vi "OLD_Dashboard Main_Fixed_1280x768.vi"() -> ()   [LabVIEW 2023]
uses:
  <vilib>/Rock Robotics/WPI/ThirdParty/JAS_Junk/TrajLib/TypeDef/FieldDisp_ElementPicture.ctl
  <vilib>/event_ctls.llb/eventvkey.ctl
  <vilib>/Rock Robotics/WPI/ThirdParty/JAS_Junk/TrajLib/Rotation2d_CreateAngle.vi
  <vilib>/Rock Robotics/WPI/ThirdParty/JAS_Junk/TrajLib/Translation2d_Create.vi
  <vilib>/Rock Robotics/WPI/ThirdParty/JAS_Junk/TrajLib/VI/FieldDisp_Element_Rotate.vi
  <vilib>/Rock Robotics/WPI/ThirdParty/JAS_Junk/TrajLib/Conv_Meters_Inches.vi
  <vilib>/Rock Robotics/WPI/ThirdParty/JAS_Junk/TrajLib/Conv_Radians_Deg.vi
  <vilib>/Rock Robotics/WPI/Dashboard/WPI_DashboardLogging Global.vi
  <vilib>/Rock Robotics/Network Tables/NT Read Boolean.vi
  <vilib>/Rock Robotics/Network Tables/NT Write Boolean.vi
  <vilib>/picture/pixmap.llb/Flatten Pixmap.vi
  <vilib>/picture/pictutil.llb/Create Mask.vi
  <vilib>/picture/picture.llb/Draw Flattened Pixmap.vi
  <vilib>/Rock Robotics/WPI/ThirdParty/JAS_Junk/TrajLib/Trajectory_Library.lvlib
panel:
  out "ROBOT":T1
  in  "Camera Settings Right":T2={"Frame Rate"=30, "Compression"=30, "Size"=1, "DB Camera Config"=FALSE} {"Frame Rate" scale=1.0..30.0; "Compression" scale=100.0..-1.0; "Size" items=["640x480", "320x240", "160x120"]}
  in  "Camera Name Right":string(combo)="No Camera Selection"
  out "Camera Perf":string
  in  "Camera Settings":T2={"Frame Rate"=30, "Compression"=30, "Size"=1, "DB Camera Config"=FALSE} {"Frame Rate" scale=1.0..30.0; "Compression" scale=100.0..-1.0; "Size" items=["640x480", "320x240", "160x120"]}
  in  "TCP":refnum<k5>
  in  "Rec Mode":enum32{"Stop", "Record", "Playback"}(radio)
  out "Robot IP":string
  out "Image Message":string="Timeout in Camera Communications"
  in  "Dashboard Tab":T3(tab)
  out "Auto Arm":bool
  out "Lower Limit Switch":bool
  out "Right Limit":bool
  out "Left Limit":bool
  out "Position":dbl
  out "Demand":dbl
  out "On Target":bool
  in  "Intake Update":bool
  in  "Shoot Update":bool
  in  "Intake":dbl
  in  "Shoot Speed":dbl
  out "State":string
  out "Misaligned":bool
  out "Have Note":bool
  out "Box Ready":bool
  out "Selected Auto":string
  out "Int Gyro Feedback":dbl
  out "Int Gyro":dbl
  in  "Update":bool
  in  "Rotation":dbl
  out "Calibrated":bool
  in  "Calibrate":bool
  in  "Select Auto":string(combo)="Select Autonomous ..."
  out "NT Connection":bool
  out "JS1 Z":dbl(slide) scale=-1.0..1.0 scale format="%#_2e"
  out "JS1 Graph":cluster{"X":dbl, "Y":dbl}[](graph)
  out "JS1 Buttons":T4
  out "JS2 Z":dbl(slide) scale=-1.0..1.0 scale format="%#_2e"
  out "JS2 Graph":cluster{"X":dbl, "Y":dbl}[](graph)
  out "JS2 Buttons":T4
  out "Mode":T5(ring)=enum."Auto Disabled"
  out "Right Camera Perf":cluster{"Bandwidth (Mbps)":dbl, "FPS":dbl}
  out "Camera Image Right":T6(plugin-control)
  out "Arm on Target":bool
  out "Velocity Deg/Sec":dbl format="%11.1f"
  out "CO":dbl format="%11.2f"
  out "PV Deg":dbl format="%11.1f"
  out "SP Deg":dbl format="%11.1f"
  out "Arm Chart":T7(graph)
  out "Right Vel":dbl format="%11.1f"
  out "Left Vel":dbl format="%11.1f"
  out "Right On Targ":bool
  out "Left On Targ":bool
  out "Right Upper (Virtual) Limit":bool
  out "Left Upper (Virtual) Limit":bool
  out "Right Low Limit":bool
  out "Right Co":dbl format="%11.2f"
  out "Right PV":dbl format="%11.1f"
  out "Left Co":dbl format="%11.2f"
  out "Left PV":dbl format="%11.1f"
  out "SP Inches":dbl format="%11.1f"
  out "Left Low Limit":bool
  out "Climb Chart":T8(graph)
  out "Left Pos":dbl
  out "Right Pos":dbl
  out "Dmd 2":dbl
  out "Right\nPosition":u8(slide) scale=0.0..14.0
  out "Left\nPosition":u8(slide) scale=0.0..14.0
  out "Dmd":u8(slide) scale=0.0..14.0
  out "Climb Blocked":bool
  out "L Mot":dbl format="%11.2f"
  out "L Speed":dbl format="%11.1f"
  out "R Mot":dbl format="%11.2f"
  out "R Speed":dbl format="%11.1f"
  out "Shoot SP\nRPM":dbl format="%11.1f"
  out "Shoot Chart":T8(graph)
  out "Robot Angle":dbl format="%11.1f"
  out "Robot Y":dbl format="%11.2f"
  out "Robot X":dbl format="%11.2f"
  out "Right April Tag Updated":bool
  out "Left April Tag Updated":bool
  out "Right Cam Connected":bool
  out "Left Cam Connected":bool
  out "Field Picture":picture
  in  "Test Slider":dbl(slide) scale=0.0..100.0 scale format="%#_3g"
  in  "On/Off":bool caption="Solenoid"
  in  "Test Name":u16(ring) items=["Select the test to run..."]
  in  "Test Tree":string(tree)
  in  "Motor":cluster{"Value":dbl, "Enable":bool} {"Value" scale=-1.0..1.0 scale format="%#_3g"}
  out "Progress":T9 {"Test Progress" scale=0.0..100.0}
  in  "Rev/Fwd":cluster{"Forward":bool, "Reverse":bool}
  in  "Test Ring":u16(ring) items=["Monochrome", "Color"]
  in  "CheckList":i32(listbox)
  out "Tree":string(tree)
  out "Camera Image":T6(plugin-control)
  in  "Camera Name":string(combo)="No Camera Selection"
  out "Background":bool
  # "HW"
  # "HW"
  # "Joysticks"
  # "Arm"
  # "Climb"
  # "Initial Rotation"
  # "Shooter & Intake"
  # "Box"
  # "Gyro"
  # "Auto"
  # "No Varible Written"
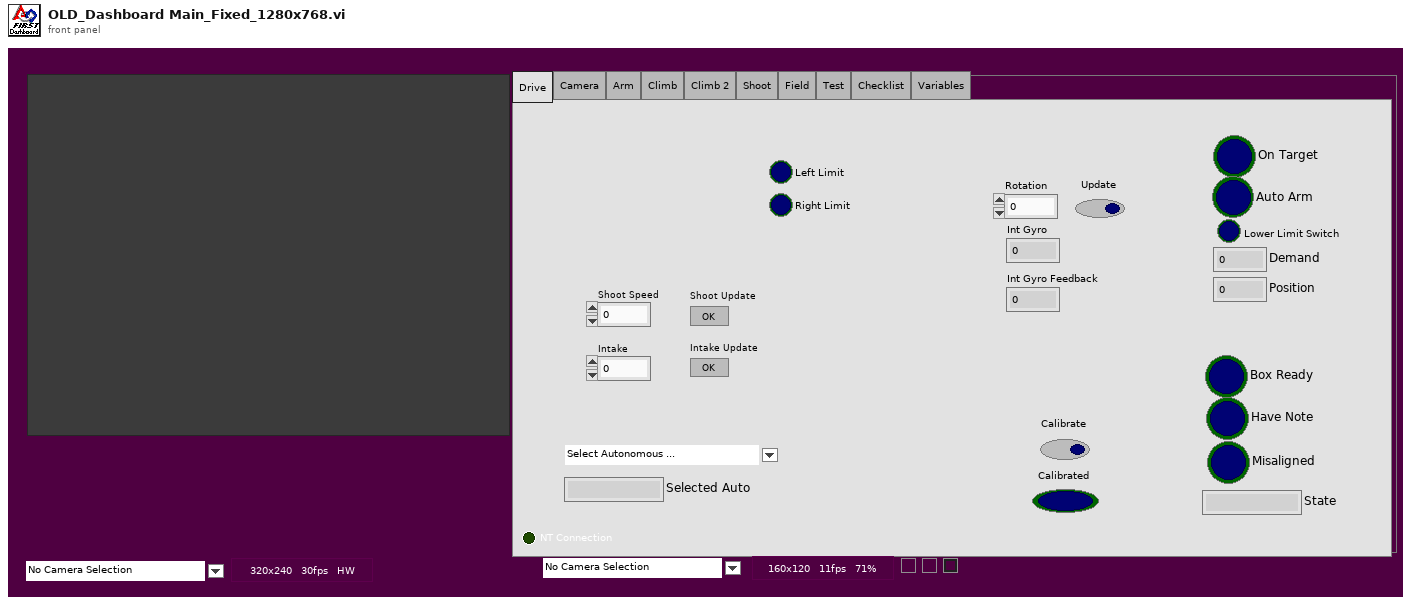
[diagram p1: front panel]
types:
  T1 = typedef "Trajectory_Library.lvlib/FieldDisp_ElementPicture.ctl" = picture
  T2 = cluster{"Frame Rate":i32, "Compression":i32, "Size":u16, "DB Camera Config":bool}
  T3 = enum32{"Drive", "Camera", "Arm", "Climb", "Climb 2", "Shoot", "Field", "Test", "Checklist", "Variables"}
  T4 = cluster{bool, bool, bool, bool, bool, bool, bool, bool, bool, bool, bool, bool}
  T5 = enum8{"Tele-Op Disabled", "Tele-Op Enabled", "Auto Disabled", "Auto Enabled", "Test Disabled", "Test Enabled", "Disconnected", "No Code", "E-Stop"}
  T6 = typedef "IMAQ Image.ctl" = refnum<image>
  T7 = cluster{"value":dbl, "value":dbl, "value":dbl, "value":dbl}
  T8 = cluster{"value":dbl, "value":dbl, "value":dbl, "value":dbl, "value":dbl}
  T9 = cluster{"Test Progress":u8, "Test Progress Text":string}
  T10 = cluster{"Save Path":path, "Interval (s)":dbl, "Keep":i32}
  T11 = enum32{"Drive", "Camera", "Basic", "Custom", "Test", "Commands", "Checklist", "Variables"}
  T12 = typedef "Image Type" = u32
  T13 = cluster{"Camera Image":refnum<vi>, "Dashboard Tab":refnum<vi>, "Background":refnum<vi>, "Rec Mode":refnum<vi>, "Test Slider":refnum<vi>, "On/Off ":refnum<vi>, "Test Ring":refnum<vi>, "Rev/Fwd":refnum<vi>, "Test Name":refnum<vi>, "Motor":refnum<vi>, "Progress":refnum<vi>, "CheckList":refnum<vi>, "Tree":refnum<vi>, "Test Tree":refnum<vi>, "Camera Settings":refnum<vi>, "Camera Name":refnum<vi>, "Camera Perf":refnum<vi>, "Camera Settings Right":refnum<vi>, "Camera Name Right":refnum<vi>, "Camera Image Right":refnum<vi>}
  T14 = cluster{"Global Rectangle":i32[], "Contours":cluster{"Contour Type":u32, "ROI Type":u32, "Points":i32[]}[]}
  T15 = cluster{"Camera Name":string, string, "Saved DB Images Info":cluster{"Save Path":path, "Interval (s)":dbl, "Keep":i32}}
  T16 = cluster{"Camera Name Right":string, string, "Saved DB Images Info":cluster{"Save Path":path, "Interval (s)":dbl, "Keep":i32}}
  T17 = cluster{"Operation":enum16{"Update", "Clear"}, "Color Box":u32}[]
  T18 = typedef "eventvkey.ctl" = enum16{"ASCII", "Enter", "Return", "Shift", "Ctrl", "Alt", "Cmd", "Opt", "Caps", "NumLock", "Clear", "Break", "Up", "Down", "Left", "Right", "Insert", "Delete", "Home", "End", "PageUp", "PageDown", "Escape", "Help", "Pause", "ScrollLock", "F1", "F2", "F3", "F4", "F5", "F6", "F7", "F8", "F9", "F10", "F11", "F12", "F13", "F14", "F15", "F16", "F17", "F18", "F19", "F20", "F21", "F22", "F23", "F24", "Play", "VolumeUp", "VolumeDown", "Mute", "Two Byte Char"}
  T19 = cluster{"Image Size":bool, "Image Type":bool, "Pixel Value":bool, "ROI Information":bool, "Zoom Factor":bool}
  T20 = cluster{"Operation":enum16{"Update", "Clear"}, "Color Box":u32}
  T21 = cluster{"Shift":bool, "Ctrl":bool, "Alt":bool, "Cmd":bool, "Opt":bool}
  T22 = typedef "Trajectory_Library.lvlib/FieldDisp_FieldElement.ctl" = cluster{"ONE-8-bit pixmap":u8[][], "Two-Array":cdb[][], "Three-Numeric":i32, "Four-Numeric":i32, "Five-Numeric":cdb, "Six-colors":u32[], "Seven-new element/subarray":u32, "Left Pixel":dbl, "Top Pixel":dbl, "Width Pix/Ft":dbl, "Height Pix/Ft":dbl, "Element Picture Ref":refnum<vi>}
  T23 = enum32{"Drive", "Camera", "Box", "Arm", "Arm 2", "Climb", "Climb 2", "Shoot", "Auto", "Field", "Vision", "Test", "Checklist", "Variables"}
  T24 = cluster{"Error Strings":string, "Disable Counts":cluster{u16, u16}, "Rail Faults":cluster{u16, u16, u16}, "Robot IP":string, "DB Mode":u8, "Event Info":cluster{"Name":string, "Type":u8, "Number":u16, "Replay":u8}}
  T25 = cluster{"Storage":cluster{"Disk Free":u64, "RAM Block":u32, "RAM free":u32}, "CPU Utilization":cluster{"CPU % ISR":sgl, "CPU % Time Crit":sgl, "CPU % Timed Str":sgl, "CPU % High":sgl, "CPU % Above":sgl, "CPU % Normal":sgl, "CPU % Low":sgl}, "CAN":cluster{"% Bus Utilization":sgl, "Bus Off Cnt":u32, "TX_FIFO Full Cnt":u32, "Receive Error Cnt":u8, "Transmit Error Cnt":u8}, "HID":cluster{"HID Outputs":u32, "Rumble Low":u16, "Rumble High":u16}[]}
  T26 = cluster{"Status bits":cluster{"Test Mode":bool, "Autonomous":bool, "Enabled":bool, "Code Start":bool, "Brownout":bool, "Reserved 2":bool, "Reserved 3":bool, "E-Stop":bool}, "Code Trace":cluster{"Disabled":bool, "TeleOp":bool, "Auto":bool, "Test":bool}, "Controller Type":enum16{"unknown", "cRIO", "roboRio"}, "Code?":enum16{"unknown", "noCode", "code"}, "Battery V":dbl}
  T27 = cluster{"Control Bits":cluster{"TestMode":bool, "Autonomous":bool, "Enabled":bool, "FMS Present":bool, bool, bool, bool, "E-Stop":bool}, "Team Station ":u8, "Countdown":sgl, "Joystick Values":cluster{"Axes":dbl[], "Buttons":bool[], "POVs":i16[]}[]}
  T28 = cluster{"Axes":dbl[], "Buttons":bool[], "POVs":i16[]}[]
  T29 = cluster{"Axes":dbl[], "Buttons":bool[], "POVs":i16[]}
  T30 = cluster{"Buttons[0]":bool, "Buttons[1]":bool, "Buttons[2]":bool, "Buttons[3]":bool, "Buttons[4]":bool, "Buttons[5]":bool, "Buttons[6]":bool, "Buttons[7]":bool, "Buttons[8]":bool, "Buttons[9]":bool, "Buttons[10]":bool, "Buttons[11]":bool}
  T31 = typedef "Trajectory_Library.lvlib/POSE2D.ctl" = cluster{"TRANSLATION":T32, "ROTATION":T33}
  T32 = typedef "Trajectory_Library.lvlib/TRANSLATION2D.ctl" = cluster{"X":dbl, "Y":dbl}
  T33 = typedef "Trajectory_Library.lvlib/ROTATION2D.ctl" = cluster{"VALUE":dbl, "COS":dbl, "SIN":dbl}
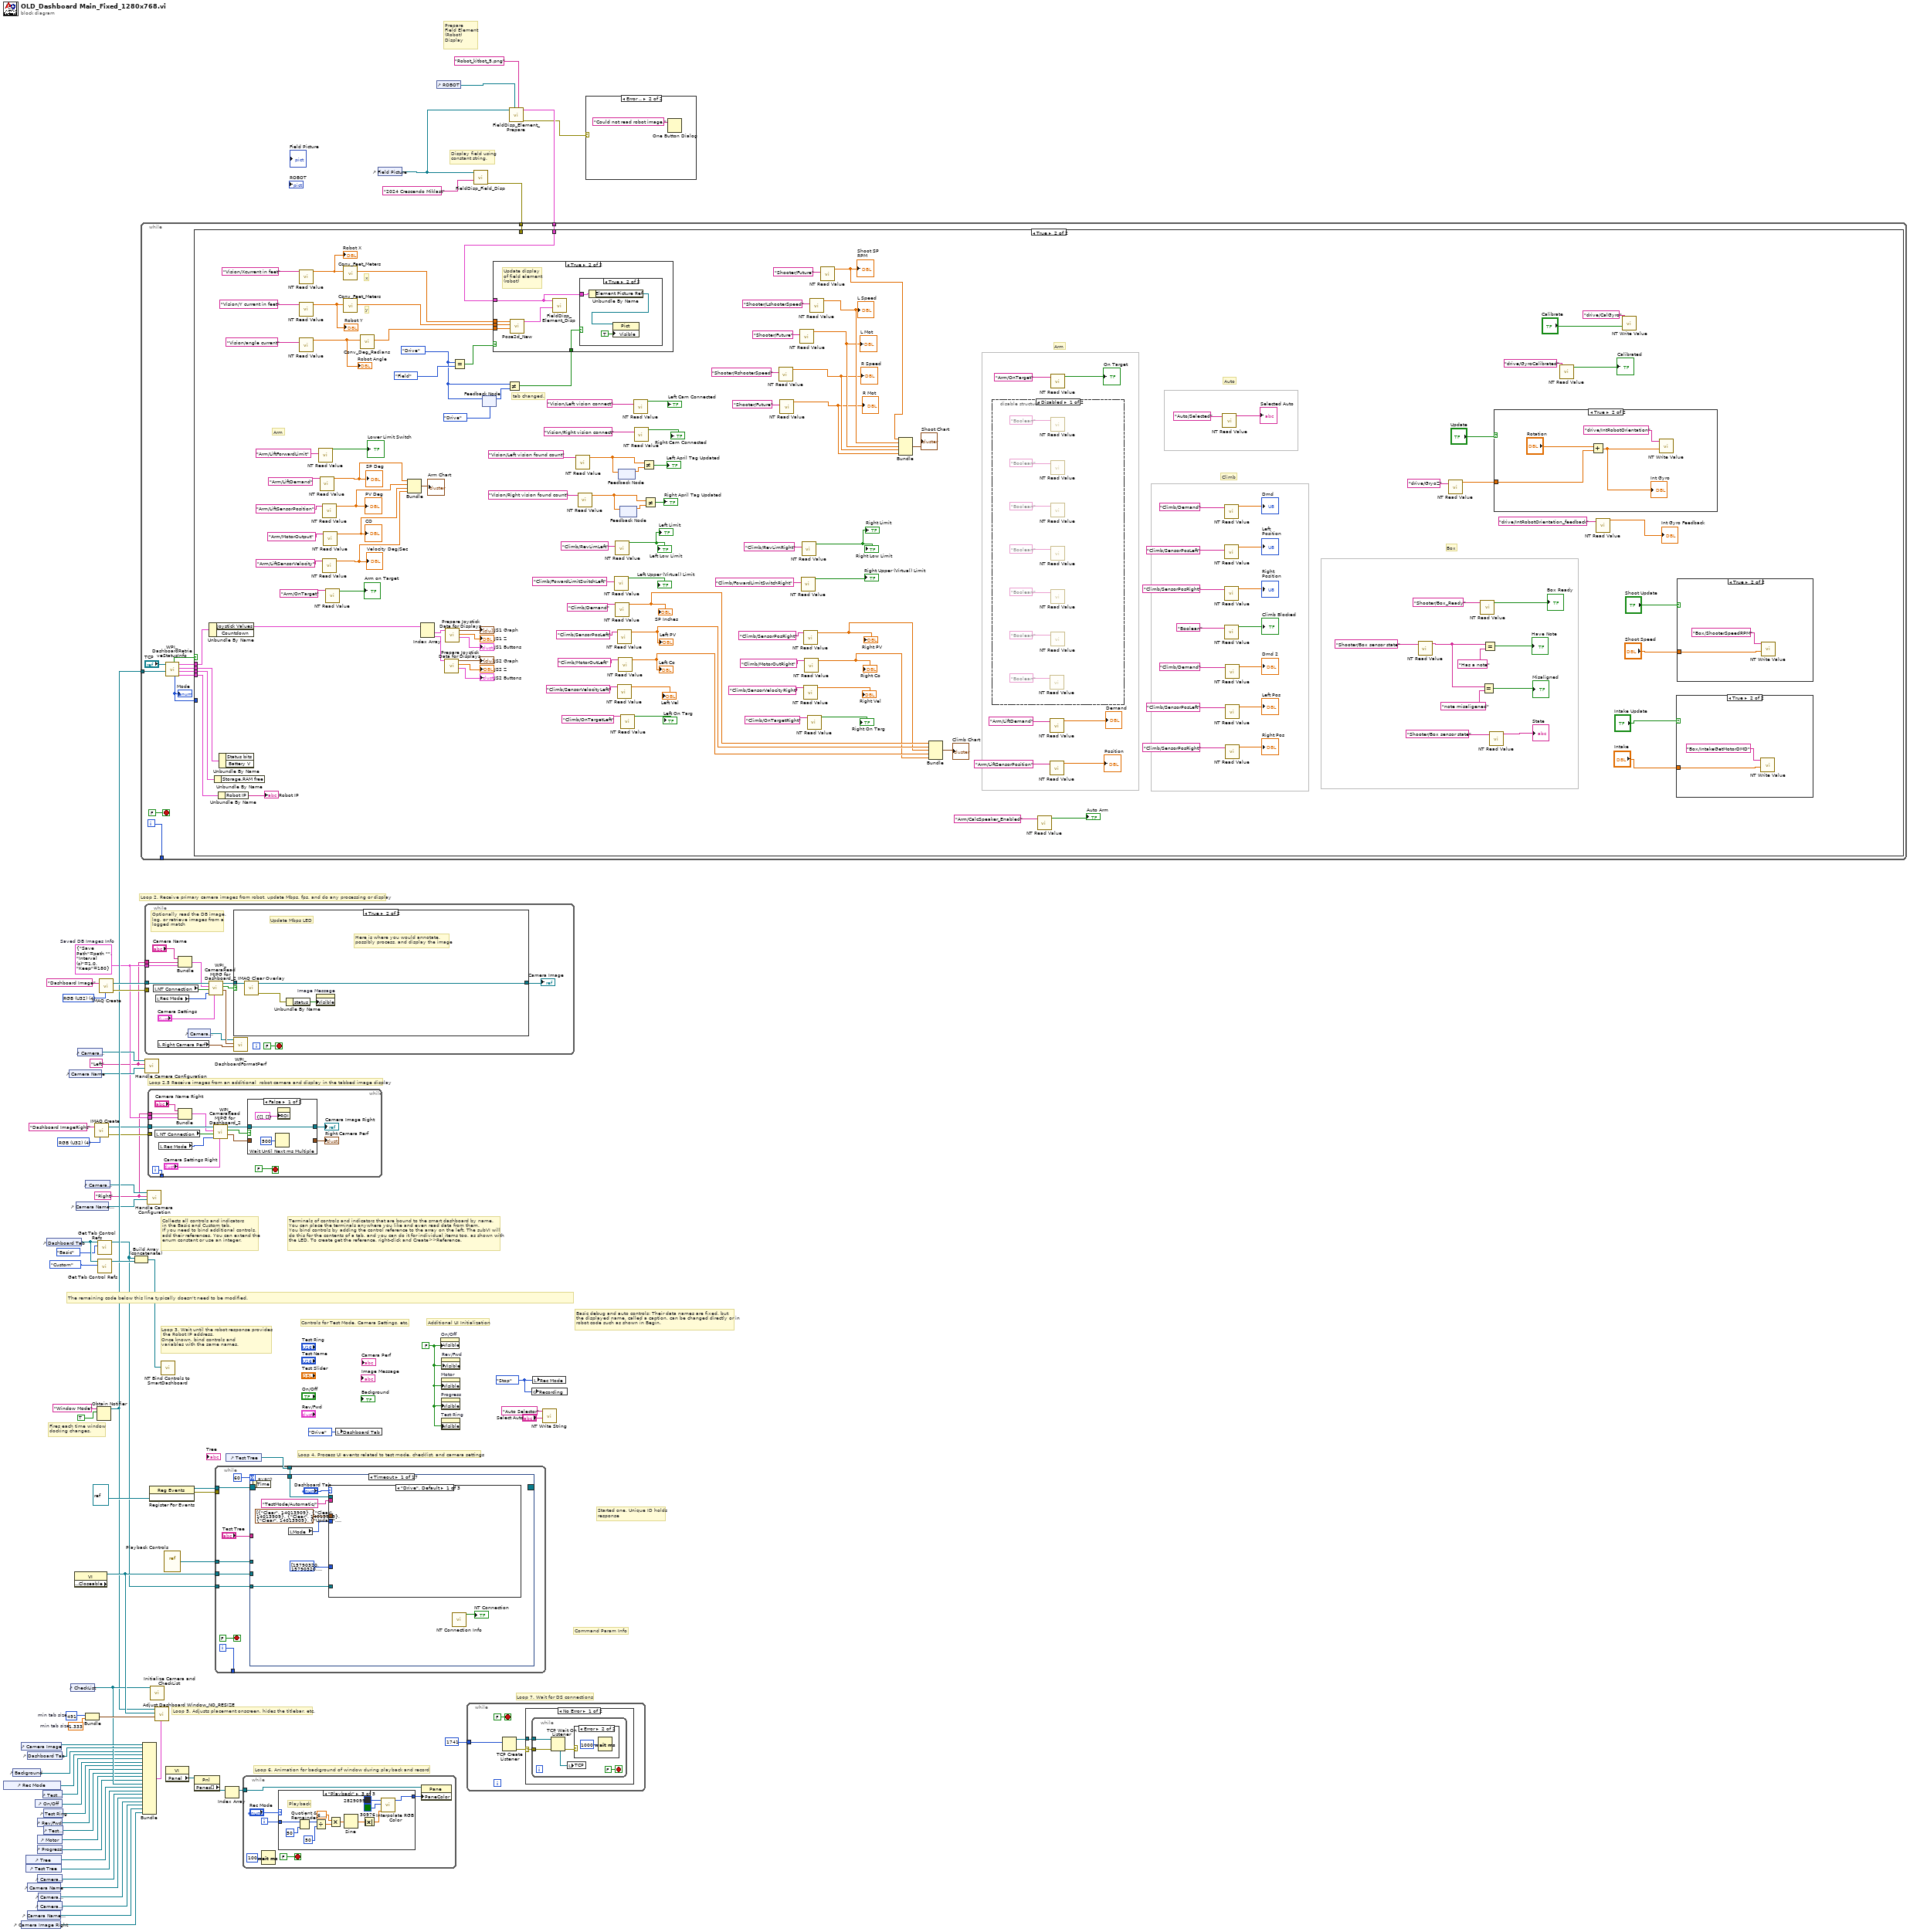
[diagram p0: block diagram]
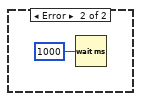
[diagram p5: hidden frame]
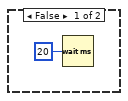
[diagram p6: hidden frame]
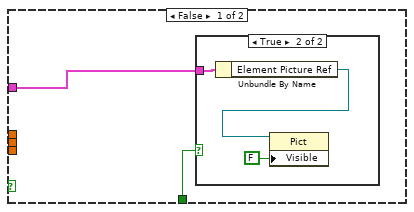
[diagram p11: hidden frame]
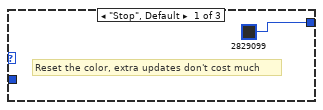
[diagram p14: hidden frame]
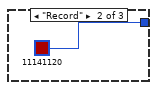
[diagram p15: hidden frame]
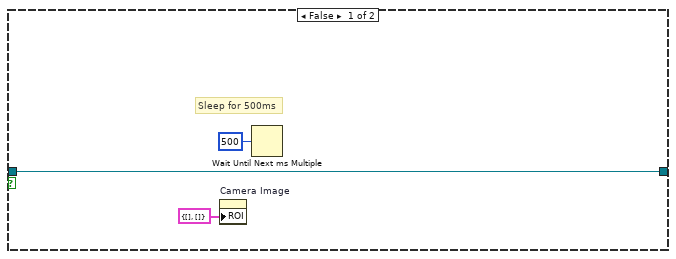
[diagram p16: hidden frame]
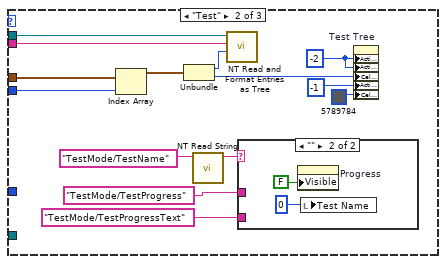
[diagram p17: hidden frame]
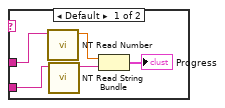
[diagram p18: hidden frame]
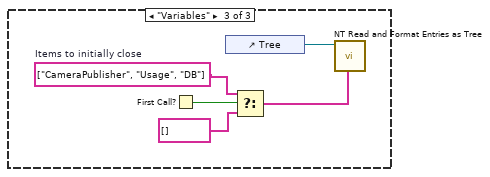
[diagram p19: hidden frame]
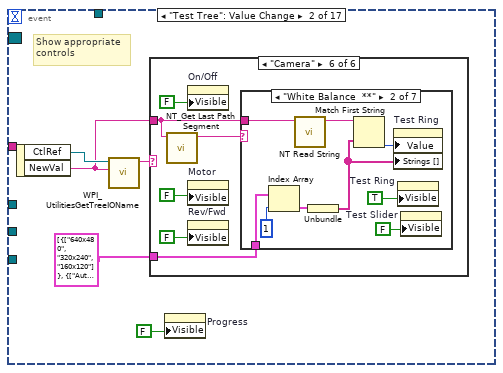
[diagram p20: hidden frame]
diagram:
  w12 = T10 {"Save Path"=path "", "Interval (s)"=1.0, "Keep"=180}  # Saved DB Images Info
  w11 = "Right"
  w10 = "Left"
  w22 = T12 4 items=["Grayscale (U8)", "Grayscale (I16)", "Grayscale (SGL)", "Complex (CSG)", "RGB (U32)", "HSL (U32)", "RGB (U64)"] ("Image Type")
  w49 = 491  # min tab size
  w48 = 1.333  # min tab size
  w56 = enum32{"Stop", "Record", "Playback"}."Stop" ("Rec Mode")
  w34 = FALSE ("Visible")
  w70 = T12 4 items=["Grayscale (U8)", "Grayscale (I16)", "Grayscale (SGL)", "Complex (CSG)", "RGB (U32)", "HSL (U32)", "RGB (U64)"] ("Image Type")
  # "Prepare\nField Element\n(Robot)\nDisplay"
  # "Display field using\nconstant string."
  # "Loop 2.5 Receive images from an additional  robot camera and display in the tabbed image display"
  # "Command Param Info"
  # "Started one, Unique ID holds\nresponse"
  # "Loop 7. Wait for DS connections"
  # "Basic debug and auto controls: Their data names are fixed, but\nthe displayed name, called a caption, can be changed directly or in\nrobot code such as shown in Begin."
  # "Controls for Test Mode, Camera Settings, etc."
  # "Additional UI Initialization"
  # "Loop 6. Animation for background of window during playback and record"
  # "Fires each time window\ndocking changes."
  # "Collects all controls and indicators\nin the Basic and Custom tab.\nIf you need to bind additional controls,\nadd their references. You can extend the\nenum constant or use an integer."
  # "The remaining code below this line typically doesn't need to be modified."
  # "Loop 4. Process UI events related to test mode, checklist, and camera settings"
  # "Terminals of controls and indicators that are bound to the smart dashboard by name.\nYou can place the terminals anywhere you like and even read data from them.\nYou bind controls by adding the control reference to the array on the left. The subVI will\ndo this for the contents of a tab, and you can do it for individual items too, as shown with\nthe LED. To create get the reference, right-click and Create>>Reference."
  # "Loop 3. Wait until the robot response provides\n the Robot IP address.\nOnce known, bind controls and\nvariables with the same names."
  # "Loop 5. Adjusts placement onscreen, hides the titlebar, etc."
  # "Loop 2. Receive primary camera images from robot, update Mbps, fps, and do any processing or display"
  n1 = control-ref of="Rec Mode"() -> (w40:refnum<vi>)
  n2 = control-ref of="Background"() -> (w9:refnum<vi>)
  n3 = control-ref of="Camera Image Right"() -> (w15:refnum<vi>)
  n4 = control-ref of="Camera Image"() -> (w51:refnum<vi>)
  n5 = control-ref of="Tree"() -> (w44:refnum<vi>)
  n6 = control-ref of="Test Tree"() -> (w43:refnum<vi>)
  n7 = control-ref of="Dashboard Tab"() -> (w50:refnum<vi>)
  n8 = control-ref of="Camera Name"() -> (w28:refnum<vi>)
  n9 = control-ref of="Camera Name Right"() -> (w16:refnum<vi>)
  n10 = control-ref of="On/Off"() -> (w38:refnum<vi>)
  n11 = control-ref of="Progress"() -> (w35:refnum<vi>)
  n12 = control-ref of="Camera Settings"() -> (w29:refnum<vi>)
  n13 = control-ref of="Camera Settings Right"() -> (w17:refnum<vi>)
  n14 = control-ref of="Rev/Fwd"() -> (w36:refnum<vi>)
  n15 = control-ref of="Motor"() -> (w41:refnum<vi>)
  n16 = control-ref of="Camera Perf"() -> (w27:refnum<vi>)
  n17 = control-ref of="Test Slider"() -> (w39:refnum<vi>)
  n18 = control-ref of="Test Ring"() -> (w37:refnum<vi>)
  n19 = control-ref of="Test Name"() -> (w42:refnum<vi>)
  n20 = control-ref of="Dashboard Tab"() -> (w54:refnum<vi>)
  n21 = control-ref of="Camera Name"() -> (w30:refnum<vi>)
  n22 = control-ref of="CheckList"() -> (w45:refnum<vi>)
  n23 = property class="VI" props=["Front Panel.Closeable"]() -> (reference out=w55:refnum<vi>)  [unwired: 2 in, 2 out]
  n24 = control-ref of="Camera Name Right"() -> (w18:refnum<vi>)
  n25 = control-ref of="Camera Settings"() -> (w31:refnum<vi>)
  n26 = control-ref of="Camera Settings Right"() -> (w19:refnum<vi>)
  n27 = Bundle("min tab size"=w49, "min tab size"=w48) -> (w47:cluster{"min tab size":i32, "min tab size":dbl})  [unwired: 1 in]
  n28 = call "IMAQ Create"("Image Name"="Dashboard ImageRight", "Image Type"=w22) -> ("New Image"=w21:T6, "error out"=w20:errorcluster)  [unwired: 2 in, 1 out]
  n29 = Obtain Notifier(name (unnamed)="Window Mode", notification data type=TRUE) -> (notifier out=w33:refnum<notifier>)  [unwired: 2 in, 2 out]
  n30 = call <vilib>:"Get Tab Control Refs.vi"("Page Index"=T11."Basic" ("Dashboard Tab"), "TabControl in"=w54) -> ("ControlsOnPage"=w26:refnum<vi>[])  [unwired: 9 in]
  n31 = call <vilib>:"Get Tab Control Refs.vi"("Page Index"=T11."Custom" ("Dashboard Tab"), "TabControl in"=w54) -> ("ControlsOnPage"=w53:refnum<vi>[])  [unwired: 9 in]
  n32 = call "IMAQ Create"("Image Name"="Dashboard Image", "Image Type"=w70) -> ("New Image"=w68:T6, "error out"=w67:errorcluster)  [unwired: 2 in, 1 out]
  n33 = Build Array (concatenate)(w26, w53) -> (w52:refnum<vi>[])
  n34 = Bundle("Camera Image"=w51, "Dashboard Tab"=w50, "Background"=w9, "Rec Mode"=w40, "Test Slider"=w39, "On/Off"=w38, "Test Ring"=w37, "Rev/Fwd"=w36, "Test Name"=w42, "Motor"=w41, "Progress"=w35, "CheckList"=w45, "Tree"=w44, "Test Tree"=w43, "Camera Settings"=w29, "Camera Name"=w28, "Camera Perf"=w27, "Camera Settings Right"=w17, "Camera Name Right"=w16, "Camera Image Right"=w15) -> (w46:T13)  [unwired: 1 in]
  n35 = call "Handle Camera Configuration.vi"("CameraNameRef"=w30, "Display Name"=w10, "ClusterRef"=w31) -> ()  [unwired: 9 in]
  n36 = while {
    tunnel: w68 -> [w84]
    tunnel: w67 -> [_]
    tunnel: w12 -> [w77]
    tunnel: w10 -> [w74]
    stop <- FALSE stop-if-true
    # "Optionally read the DB image,\nlog, or retrieve images from a\nlogged match"
    n37 = local read "NT Connection"() -> (w78:bool)
    n38 = local read "Rec Mode"() -> (w81:enum32{"Stop", "Record", "Playback"})
    n39 = local read "Right Camera Perf"() -> (w72:cluster{"Bandwidth (Mbps)":dbl, "FPS":dbl})
    n40 = Bundle("Camera Name"="Camera Name", w74, "Saved DB Images Info"=w77) -> (w76:T15)  [unwired: 1 in]
    n41 = control-ref of="Camera Perf"() -> (w71:refnum<vi>)
    n42 = call <vilib>:"WPI_CameraRead MJPG for Dashboard_2.vi"("Camera Settings"="Camera Settings", "Rec Mode"=w81, "NT Connection"=w78, "Capture Info"=w76, "Image in"=w84) -> ("perf info"=w73:cluster{"Bandwidth (Mbps)":dbl, "fps":dbl}, "Active"=w82:bool, "Image\\ out"=w83:T6)  [unwired: 4 in]
    n43 = case shown="True" w82 {
      tunnel: w83 -> [w87 w90]
      tunnel: [w87 w89] -> w79
      frame False {
        # "Sleep for 500ms"
        n44 = property on="Camera Image" class="ImageControl"("ROI"=T14 {"Global Rectangle"=[], "Contours"=[]}) -> ()  [unwired: 2 in, 2 out]
        n45 = Wait Until Next ms Multiple(millisecond multiple=u32 500) -> ()  [unwired: 1 out]
      }
      frame True {
        # "Here is where you would annotate,\npossibly process, and display the image"
        # "Update Mbps LED"
        n46 = call "IMAQ Clear Overlay"("Image"=w90) -> ("error out"=w91:errorcluster, "Image Out"=w89:T6)  [unwired: 2 in, 7 out]
        n47 = Unbundle By Name(w91) -> ("status"=w92:bool)
        n48 = property on="Image Message" class="Str"("Visible"=w92) -> ()  [unwired: 2 in, 2 out]
      }
    }
    "Camera Image" <- w79
    n49 = call <vilib>:"WPI_DashboardFormatPerf.vi"("Right Camera Perf"=w72, "Performance"=w73, "String in"=w71) -> ()  [unwired: 9 in]
  }
  n50 = call "Handle Camera Configuration.vi"("CameraNameRef"=w18, "Display Name"=w11, "ClusterRef"=w19) -> ()  [unwired: 9 in]
  n51 = while {
    tunnel: w21 -> [w107]
    tunnel: w20 -> [_]
    tunnel: [w102] -> _
    tunnel: w12 -> [w98]
    tunnel: w11 -> [w95]
    i -> [w102]
    stop <- FALSE stop-if-true
    n52 = local read "NT Connection"() -> (w99:bool)
    n53 = local read "Rec Mode"() -> (w106:enum32{"Stop", "Record", "Playback"})
    n54 = Bundle("Camera Name Right"="Camera Name Right", w95, "Saved DB Images Info"=w98) -> (w97:T16)  [unwired: 1 in]
    n55 = call <vilib>:"WPI_CameraRead MJPG for Dashboard_2.vi"("Camera Settings"="Camera Settings Right", "Rec Mode"=w106, "NT Connection"=w99, "Capture Info"=w97, "Image in"=w107) -> ("perf info"=w93:cluster{"Bandwidth (Mbps)":dbl, "fps":dbl}, "Active"=w101:bool, "Image\\ out"=w104:T6)  [unwired: 4 in]
    n56 = case shown="False" w101 {
      tunnel: w104 -> [w109 w112]
      tunnel: [w109 w112] -> w100
      tunnel: [_ w111] -> w94
      tunnel: w93 -> [_ w111]
      frame False {
        n57 = Wait Until Next ms Multiple(millisecond multiple=u32 500) -> ()  [unwired: 1 out]
        n58 = property on="Camera Image Right" class="ImageControl"("ROI"=T14 {"Global Rectangle"=[], "Contours"=[]}) -> ()  [unwired: 2 in, 2 out]
      }
      frame True {
      }
    }
    "Camera Image Right" <- w100
    "Right Camera Perf" <- w94
  }
  n59 = register-events(refnum<vi> refnum) -> (reference out=w59:refnum<event-registration>, error out=w58:errorcluster)  [unwired: 2 in]
  n60 = call "Initialize Camera and CheckList.vi"("ListBox in"=w45) -> ()  [unwired: 11 in]
  n61 = call "Adjust Dashboard Window_NO_RESIZE.vi"("Sizing Refnums"=w46, "Size Constraints"=w47, "VI"=w55, "WIn Mode"=w33) -> ()  [unwired: 8 in]
  n62 = call <vilib>:"NT Bind Controls to SmartDashboard.vi"("Bound Control Refs"=w52) -> ()  [unwired: 11 in]
  n63 = vi-ref "Playback Controls.vi"() -> (w60:refnum<vi>)
  n64 = property class="VI"() -> ("Panel"=w62:refnum<vi>)  [unwired: 2 in, 2 out]
  n65 = property class="Pnl"(reference=w62) -> ("Panes[]"=w63:refnum<vi>[])  [unwired: 1 in, 2 out]
  n66 = Index Array(array=w63) -> (element=w61:refnum<vi>)  [unwired: 1 in]
  n67 = control-ref of="Test Tree"() -> (w64:refnum<vi>)
  n68 = while {
    tunnel: [w118] -> _
    tunnel: w64 -> [w117]
    tunnel: w60 -> [w116]
    tunnel: w59 -> [w115]
    tunnel: w58 -> [_]
    tunnel: w55 -> [w114]
    tunnel: w26 -> [w113]
    i -> [w118]
    stop <- FALSE stop-if-true
    n69 = event shown="[0] Timeout" {
      selector: w115 -> [_ _ _ _ _ _ _ _ _ _ _ _ _ _ _ _ _]
      dyn-events: [_ _ _ _ _ _ _ _ _ _ _ _ _ w322 _ _ _] -> _
      timeout: u32 60 ("milliseconds to wait") -> [_ _ _ _ _ _ _ _ _ _ _ _ _ _ _ _ _]
      tunnel: w117 -> [w128 _ _ _ _ _ _ _ _ _ _ _ _ _ _ _ _]
      tunnel: "Test Tree" -> [_ _ _ _ _ _ _ _ w295 w302 w303 w306 w313 _ _ _ _]
      tunnel: w116 -> [_ _ _ _ _ _ _ _ _ _ _ _ _ w324 _ w339 _]
      tunnel: w114 -> [_ _ _ _ _ _ _ _ _ _ _ _ _ w320 _ _ _]
      tunnel: w113 -> [w123 _ _ _ _ _ _ _ _ _ _ _ _ _ _ _ _]
      event Timeout {
        n70 = event-data() -> ()  [unwired: 1 in, 1 out]
        n71 = local read "Mode"() -> (w126:T5)
        n72 = case shown="\"Drive\", Default" "Dashboard Tab" {
          tunnel: w128 -> [_ w143 _]
          tunnel: "TestMode/Automatic/" ("Name Pattern") -> [_ w142 _]
          tunnel: T17 [{"Operation"=enum."Clear", "Color Box"=14013909}, {"Operation"=enum."Clear", "Color Box"=14013909}, {"Operation"=enum."Clear", "Color Box"=14013909}, {"Operation"=enum."Clear", "Color Box"=14013909}, {"Operation"=enum."Update", "Color Box"=14013909}, {"Operation"=enum."Update", "Color Box"=16777215}, {"Operation"=enum."Clear", "Color Box"=14013909}, {"Operation"=enum."Clear", "Color Box"=14013909}, {"Operation"=enum."Clear", "Color Box"=14013909}] -> [_ w135 _]
          tunnel: w126 -> [_ w134 _]
          tunnel: u32[] [15790320, 15790320, 15790320, 15790320, 16777215, 16777215, 15790320, 15790320, 15790320] -> [_ _ _]
          tunnel: w123 -> [_ _ _]
          frame "Drive", Default {
          }
          frame "Test" {
            w141 = -2 ("Active Item:Row Number")
            n73 = Index Array(array=w135, index=w134) -> (element=w136:T20)
            n74 = Unbundle(w136) -> ("Operation"=w137:enum16{"Update", "Clear"}, "Color Box"=w138:u32)
            n75 = call <vilib>:"NT Read String.vi"("name"="TestMode/TestName" ("Name")) -> ("value"=w132:string)  [unwired: 8 in, 2 out]
            n76 = call <vilib>:"NT Read and Format Entries as Tree.vi"("Operation"=w137, "Name Pattern"=w142, "Tree Refnum"=w143) -> ()  [unwired: 7 in, 2 out]
            n77 = case shown="\"\"" w132 {
              tunnel: "TestMode/TestProgress" ("Name") -> [w145 _]
              tunnel: "TestMode/TestProgressText" ("Name") -> [w144 _]
              frame Default {
                n78 = call <vilib>:"NT Read Number.vi"("name"=w145) -> ("value"=w146:dbl)  [unwired: 8 in, 2 out]
                n79 = call <vilib>:"NT Read String.vi"("name"=w144) -> ("value"=w147:string)  [unwired: 8 in, 2 out]
                n80 = Bundle("value"=w146, "value"=w147) -> (→"Progress":cluster{"value":dbl, "value":string})  [unwired: 1 in]
              }
              frame "" {
                n81 = property on="Progress" class="Clust (strict)"("Visible"=FALSE) -> ()  [unwired: 2 in, 2 out]
                n82 = local write "Test Name"(u16 0) -> ()
              }
            }
            n83 = property on="Test Tree" class="Tree (strict)"("Active Item Row Number"=w141, "ActiveColNum"=w141, "CellBG"=w138, "Active Item Row Number"=-1 ("Active Item:Row Number"), "CellBG"=u32 5789784 ("Color Box")) -> ()  [unwired: 2 in, 2 out]
          }
          frame "Variables" {
            w153 = string[] ["CameraPublisher", "Usage", "DB"]  # Items to initially close
            n84 = First Call?() -> (First Call?: T/F=w154:bool)
            n85 = control-ref of="Tree"() -> (w155:refnum<vi>)
            n86 = Select(t=w153, s=w154, f=string[] []) -> (s? t:f=w151:string[])
            n87 = call <vilib>:"NT Read and Format Entries as Tree.vi"("Tags to  Close"=w151, "Tree Refnum"=w155) -> ()  [unwired: 8 in, 2 out]
          }
        }
        n88 = call <vilib>:"NT Connection Info.vi"() -> ("Connected"=→"NT Connection":bool)  [unwired: 11 in]
      }
      event "Test Tree": Value Change {
        # "Show appropriate\ncontrols"
        n89 = event-data() -> ("CtlRef"=w159:refnum<vi>, "NewVal"=w157:string)  [unwired: 1 in]
        n90 = call <vilib>:"WPI_UtilitiesGetTreeIOName.vi"("NewVal"=w157, "TreeControl in"=w159) -> ("I/O Name"=w160:string)  [unwired: 9 in]
        n91 = case shown="\"Camera\"" w160 {
          selector: w160 -> [_ w167 _ w189 w198 _]
          tunnel: w157 -> [_ _ w186 w188 _ w205]
          tunnel: cluster{string[]}[] [{["640x480", "320x240", "160x120"]}, {["Auto", "Fixed indoor", "Fixed outdoor 1", "Fixed outdoor 2", "Fixed fluorescent 1", "Fixed fluorescent 2", "Hold current"]}, {["Auto", "Flicker-free 50 Hz", "Flicker-free 60 Hz", "Hold current"]}, {["None", "Prioritize frame rate", "Prioritize image quality"]}, {["Monochrome", "Color"]}] -> [_ _ _ _ _ w204]
          frame Default {
            w162 = FALSE ("Visible")
            w161 = FALSE ("Visible")
            n92 = property on="Motor" class="Clust (strict)"("Visible"=w161) -> ()  [unwired: 2 in, 2 out]
            n93 = property on="Test Ring" class="Ring (strict)"("Visible"=w161) -> ()  [unwired: 2 in, 2 out]
            n94 = property on="Rev/Fwd" class="Clust (strict)"("Visible"=w162) -> ()  [unwired: 2 in, 2 out]
            n95 = property on="On/Off" class="Bool (strict)"("Visible"=w162) -> ()  [unwired: 2 in, 2 out]
            n96 = property on="Test Slider" class="Slide (strict)"("Visible"=w162) -> ()  [unwired: 2 in, 2 out]
          }
          frame "Analog Out", "Motor", "PWM" {
            w168 = FALSE ("Visible")
            n97 = case shown="\"Analog Out\"" w167 {
              tunnel: [1.0 ("Value") -1.0 ("Value") 0.0 ("Value")] -> w166
              tunnel: [255.0 ("Value") 1.0 ("Value") 5.0 ("Value")] -> w165
              tunnel: [128.0 ("Value") 0.0 ("Value") 0.0 ("Value")] -> w164
              tunnel: [64.0 ("Value") 0.5 ("Value") 1.0 ("Value")] -> w163
              frame "PWM" {
              }
              frame "Motor", Default {
              }
              frame "Analog Out" {
              }
            }
            n98 = property on="Motor" class="Clust (strict)"("Visible"=TRUE) -> ()  [unwired: 2 in, 2 out]
            n99 = property on="Value" class="Slide (strict)"("Value"=w164, "Scale.Minimum"=w166, "Scale.Maximum"=w165, "Scale.Increment"=w163) -> ()  [unwired: 2 in, 2 out]
            n100 = property on="On/Off" class="Bool (strict)"("Visible"=w168) -> ()  [unwired: 2 in, 2 out]
            n101 = property on="Test Slider" class="Slide (strict)"("Visible"=w168) -> ()  [unwired: 2 in, 2 out]
            n102 = property on="Test Ring" class="Ring (strict)"("Visible"=w168) -> ()  [unwired: 2 in, 2 out]
            n103 = property on="Rev/Fwd" class="Clust (strict)"("Visible"=w168) -> ()  [unwired: 2 in, 2 out]
          }
          frame "Servo" {
            w184 = FALSE ("Visible")
            n104 = call <vilib>:"NT Read Number.vi"("name"=w186) -> ("value"=w185:dbl)  [unwired: 8 in, 2 out]
            n105 = property on="Test Slider" class="Slide (strict)"("Visible"=TRUE, "Scale.Maximum"=170.0 ("Scale.Range:Maximum")) -> ()  [unwired: 2 in, 2 out]
            n106 = local write "Test Slider"(w185) -> ()
            n107 = property on="Motor" class="Clust (strict)"("Visible"=w184) -> ()  [unwired: 2 in, 2 out]
            n108 = property on="Rev/Fwd" class="Clust (strict)"("Visible"=w184) -> ()  [unwired: 2 in, 2 out]
            n109 = property on="On/Off" class="Bool (strict)"("Visible"=w184) -> ()  [unwired: 2 in, 2 out]
            n110 = property on="Test Ring" class="Ring (strict)"("Visible"=w184) -> ()  [unwired: 2 in, 2 out]
          }
          frame "Relay", "Solenoid" {
            w187 = FALSE ("Visible")
            n111 = property on="Motor" class="Clust (strict)"("Visible"=w187) -> ()  [unwired: 2 in, 2 out]
            n112 = property on="Test Slider" class="Slide (strict)"("Visible"=w187) -> ()  [unwired: 2 in, 2 out]
            n113 = Search and Replace String(input string=w188, search string="/Value  **", replace string="/Direction") -> (result string=w194:string)  [unwired: 5 in, 3 out]
            n114 = property on="Test Ring" class="Ring (strict)"("Visible"=w187) -> ()  [unwired: 2 in, 2 out]
            n115 = call <vilib>:"NT Read String.vi"("name"=w194) -> ("value"=w192:string)  [unwired: 8 in, 2 out]
            n116 = Equal?(x="Both directions", y=w192) -> (x = y?=w190:bool)
            n117 = Not(x=w190) -> (.not. x?=w191:bool)
            n118 = property on="Rev/Fwd" class="Clust (strict)"("Visible"=w190) -> ()  [unwired: 2 in, 2 out]
            n119 = property on="On/Off" class="Bool (strict)"("Visible"=w191, "Caption.Text"=w189) -> ()  [unwired: 2 in, 2 out]
          }
          frame "Compressor", "Digital Out" {
            w197 = FALSE ("Visible")
            # "Get direction and finish"
            n120 = property on="Motor" class="Clust (strict)"("Visible"=w197) -> ()  [unwired: 2 in, 2 out]
            n121 = property on="Test Slider" class="Slide (strict)"("Visible"=w197) -> ()  [unwired: 2 in, 2 out]
            n122 = property on="Test Ring" class="Ring (strict)"("Visible"=w197) -> ()  [unwired: 2 in, 2 out]
            n123 = property on="On/Off" class="Bool (strict)"("Visible"=TRUE, "Caption.Text"=w198) -> ()  [unwired: 2 in, 2 out]
            n124 = property on="Rev/Fwd" class="Clust (strict)"("Visible"=FALSE) -> ()  [unwired: 2 in, 2 out]
          }
          frame "Camera" {
            n125 = call <vilib>:"NT_Get Last Path Segment.vi"("String in"=w205) -> ("String out"=w206:string)  [unwired: 10 in]
            n126 = property on="On/Off" class="Bool (strict)"("Visible"=FALSE) -> ()  [unwired: 2 in, 2 out]
            n127 = property on="Motor" class="Clust (strict)"("Visible"=FALSE) -> ()  [unwired: 2 in, 2 out]
            n128 = property on="Rev/Fwd" class="Clust (strict)"("Visible"=FALSE) -> ()  [unwired: 2 in, 2 out]
            n129 = case shown="\"White Balance  **\"" w206 {
              tunnel: w205 -> [w212 w221 w230 w239 w248 _ w254]
              tunnel: w204 -> [w210 w218 w227 w236 w245 _ _]
              frame "Size  **" {
                n130 = Index Array(array=w210) -> (element=w209:cluster{string[]})  [unwired: 1 in]
                n131 = call <vilib>:"NT Read String.vi"("name"=w212) -> ("value"=w211:string)  [unwired: 8 in, 2 out]
                n132 = Unbundle(w209) -> (w207:string[])
                n133 = Match First String(2:w207, 3:w211) -> (0:w208:i32)  [unwired: 1 out]
                n134 = property on="Test Ring" class="Ring (strict)"("Value"=w208, "Strings []"=w207) -> ()  [unwired: 2 in, 2 out]
                n135 = property on="Test Ring" class="Ring (strict)"("Visible"=TRUE) -> ()  [unwired: 2 in, 2 out]
                n136 = property on="Test Slider" class="Slide (strict)"("Visible"=FALSE) -> ()  [unwired: 2 in, 2 out]
              }
              frame "White Balance  **" {
                n137 = Index Array(array=w218, index=1) -> (element=w219:cluster{string[]})
                n138 = call <vilib>:"NT Read String.vi"("name"=w221) -> ("value"=w220:string)  [unwired: 8 in, 2 out]
                n139 = Unbundle(w219) -> (w216:string[])
                n140 = Match First String(2:w216, 3:w220) -> (0:w215:i32)  [unwired: 1 out]
                n141 = property on="Test Ring" class="Ring (strict)"("Value"=w215, "Strings []"=w216) -> ()  [unwired: 2 in, 2 out]
                n142 = property on="Test Ring" class="Ring (strict)"("Visible"=TRUE) -> ()  [unwired: 2 in, 2 out]
                n143 = property on="Test Slider" class="Slide (strict)"("Visible"=FALSE) -> ()  [unwired: 2 in, 2 out]
              }
              frame "Exposure  **" {
                n144 = Index Array(array=w227, index=2) -> (element=w228:cluster{string[]})
                n145 = call <vilib>:"NT Read String.vi"("name"=w230) -> ("value"=w229:string)  [unwired: 8 in, 2 out]
                n146 = Unbundle(w228) -> (w224:string[])
                n147 = Match First String(2:w224, 3:w229) -> (0:w225:i32)  [unwired: 1 out]
                n148 = property on="Test Ring" class="Ring (strict)"("Value"=w225, "Strings []"=w224) -> ()  [unwired: 2 in, 2 out]
                n149 = property on="Test Ring" class="Ring (strict)"("Visible"=TRUE) -> ()  [unwired: 2 in, 2 out]
                n150 = property on="Test Slider" class="Slide (strict)"("Visible"=FALSE) -> ()  [unwired: 2 in, 2 out]
              }
              frame "Exposure Priority  **" {
                n151 = Index Array(array=w236, index=3) -> (element=w237:cluster{string[]})
                n152 = call <vilib>:"NT Read String.vi"("name"=w239) -> ("value"=w238:string)  [unwired: 8 in, 2 out]
                n153 = Unbundle(w237) -> (w233:string[])
                n154 = Match First String(2:w233, 3:w238) -> (0:w234:i32)  [unwired: 1 out]
                n155 = property on="Test Ring" class="Ring (strict)"("Value"=w234, "Strings []"=w233) -> ()  [unwired: 2 in, 2 out]
                n156 = property on="Test Ring" class="Ring (strict)"("Visible"=TRUE) -> ()  [unwired: 2 in, 2 out]
                n157 = property on="Test Slider" class="Slide (strict)"("Visible"=FALSE) -> ()  [unwired: 2 in, 2 out]
              }
              frame "Color Enable  **" {
                n158 = Index Array(array=w245, index=4) -> (element=w246:cluster{string[]})
                n159 = call <vilib>:"NT Read String.vi"("name"=w248) -> ("value"=w247:string)  [unwired: 8 in, 2 out]
                n160 = Unbundle(w246) -> (w242:string[])
                n161 = Match First String(2:w242, 3:w247) -> (0:w243:i32)  [unwired: 1 out]
                n162 = property on="Test Ring" class="Ring (strict)"("Value"=w243, "Strings []"=w242) -> ()  [unwired: 2 in, 2 out]
                n163 = property on="Test Ring" class="Ring (strict)"("Visible"=TRUE) -> ()  [unwired: 2 in, 2 out]
                n164 = property on="Test Slider" class="Slide (strict)"("Visible"=FALSE) -> ()  [unwired: 2 in, 2 out]
              }
              frame Default {
                n165 = property on="Test Ring" class="Ring (strict)"("Visible"=FALSE) -> ()  [unwired: 2 in, 2 out]
                n166 = property on="Test Slider" class="Slide (strict)"("Visible"=FALSE) -> ()  [unwired: 2 in, 2 out]
              }
              frame "Brightness  **", "Color Level  **", "Compression  **", "FPS  **", "Sharpness  **" {
                n167 = call <vilib>:"NT Read Number.vi"("name"=w254) -> ("value"=w253:dbl)  [unwired: 8 in, 2 out]
                n168 = local write "Test Slider"(w253) -> ()
                n169 = property on="Test Ring" class="Ring (strict)"("Visible"=FALSE) -> ()  [unwired: 2 in, 2 out]
                n170 = property on="Test Slider" class="Slide (strict)"("Visible"=TRUE, "Scale.Maximum"=100.0 ("Scale.Range:Maximum")) -> ()  [unwired: 2 in, 2 out]
              }
            }
          }
        }
        n171 = property on="Progress" class="Clust (strict)"("Visible"=FALSE) -> ()  [unwired: 2 in, 2 out]
      }
      event "Test Name": Mouse Enter {
        # "Populate the ring with the list of tests"
        n172 = event-data() -> ()  [unwired: 1 in, 1 out]
        n173 = call <vilib>:"NT Read String Array.vi"("name"="TestMode/TestList" ("Name")) -> ("value"=w261:string[])  [unwired: 8 in, 2 out]
        n174 = Build Array (concatenate)("Select the test to run...", w261) -> (w260:string[])
        n175 = property on="Test Name" class="Ring (strict)"("Strings []"=w260) -> ()  [unwired: 2 in, 2 out]
      }
      event "Test Name": Value Change {
        w262 = FALSE ("Visible")
        # "Tell the robot the test name to run"
        n176 = event-data() -> ("NewVal"=w266:u16)  [unwired: 1 in]
        n177 = property on="Test Name" class="Ring (strict)"() -> ("Strings []"=w267:string[])  [unwired: 2 in, 2 out]
        n178 = local write "Progress"(T9 {"Test Progress"=0, "Test Progress Text"=""} ("Progress")) -> ()
        n179 = Index Array(array=w267, index=w266) -> (element=w265:string)
        n180 = call <vilib>:"NT Write String.vi"("value"=w265, "name"="TestMode/TestName" ("Name")) -> ()  [unwired: 9 in, 1 out]
        n181 = property on="Progress" class="Clust (strict)"("Visible"=TRUE) -> ()  [unwired: 2 in, 2 out]
        n182 = property on="Motor" class="Clust (strict)"("Visible"=w262) -> ()  [unwired: 2 in, 2 out]
        n183 = property on="Test Slider" class="Slide (strict)"("Visible"=w262) -> ()  [unwired: 2 in, 2 out]
        n184 = property on="On/Off" class="Bool (strict)"("Visible"=w262) -> ()  [unwired: 2 in, 2 out]
        n185 = property on="Rev/Fwd" class="Clust (strict)"("Visible"=w262) -> ()  [unwired: 2 in, 2 out]
        n186 = property on="Test Ring" class="Ring (strict)"("Visible"=w262) -> ()  [unwired: 2 in, 2 out]
      }
      event "Select Auto": Mouse Enter {
        # "Populate the combo box with the list of autonomous options"
        n187 = event-data() -> ()  [unwired: 1 in, 1 out]
        n188 = call <vilib>:"NT Read String Array.vi"("name"="Auto List" ("Name")) -> ("value"=w269:string[])  [unwired: 8 in, 2 out]
        n189 = property on="Select Auto" class="CmbBox"("Strings[]"=w269) -> ()  [unwired: 2 in, 2 out]
      }
      event "Select Auto": Value Change {
        # "User modified the Auto Selection. Write to NT variable so robot knows."
        n190 = event-data() -> ("NewVal"=w271:string)  [unwired: 1 in]
        n191 = call <vilib>:"NT Write String.vi"("value"=w271, "name"="Auto Selector" ("Name")) -> ()  [unwired: 9 in, 1 out]
      }
      event "CheckList": Double Click {
        # "Shift clears all"
        # "Update symbols on the listbox"
        n192 = event-data() -> ("PlatMods.Shift"=w273:bool, "Row"=w275:i32)  [unwired: 1 in]
        n193 = case shown="True" w273 {
          tunnel: w275 -> [w279 _]
          tunnel: 1 -> [w278 _]
          frame False {
            n194 = property on="CheckList" class="LstBox (strict)"() -> ("Item Symbols"=w277:i32[])  [unwired: 2 in, 2 out]
            n195 = Replace Array Subset(array=w277, new element=w278, index=w279) -> (w276:i32[])
            n196 = property on="CheckList" class="LstBox (strict)"("Item Symbols"=w276) -> ()  [unwired: 2 in, 2 out]
          }
          frame True {
            w280 = 0 ("Top Row")
            n197 = property on="CheckList" class="LstBox (strict)"() -> ("Number of Rows"=w282:u32)  [unwired: 2 in, 2 out]
            n198 = Initialize Array(0, w282) -> (w281:i32[])
            n199 = property on="CheckList" class="LstBox (strict)"("Top Row"=w280, "Value"=w280, "Item Symbols"=w281) -> ()  [unwired: 2 in, 2 out]
          }
        }
      }
      event "CheckList": Key Down {
        # "Update symbols on the listbox\nLeft and right keys check and uncheck"
        n200 = event-data() -> ("VKey"=w285:T18)  [unwired: 1 in]
        n201 = case shown="\"Left\", \"Right\"" w285 {
          selector: w285 -> [w290 _]
          tunnel: eventvkey."Left" ("VKey") -> [w288 _]
          frame "Left", "Right" {
            n202 = Equal?(x=w288, y=w290) -> (x = y?=w289:bool)
            n203 = Select(t=0, s=w289, f=1) -> (s? t:f=w291:i32)
            n204 = property on="CheckList" class="LstBox (strict)"() -> ("Item Symbols"=w294:i32[])  [unwired: 2 in, 2 out]
            n205 = Replace Array Subset(array=w294, new element=w291, index="CheckList") -> (w293:i32[])
            n206 = property on="CheckList" class="LstBox (strict)"("Item Symbols"=w293) -> ()  [unwired: 2 in, 2 out]
          }
          frame Default {
          }
        }
      }
      event "Motor.Enable": Value Change {
        # "When the test mode otor enable helper is set, update that\ntree row item's value"
        n207 = event-data() -> ("NewVal"=w299:bool)  [unwired: 1 in]
        n208 = Unbundle("Motor") -> ("Value"=w298:dbl)  [unwired: 1 out]
        n209 = Select(t=w298, s=w299, f=0.0) -> (s? t:f=w296:dbl)
        n210 = call <vilib>:"NT Write Number.vi"("value"=w296, "name"=w295) -> ()  [unwired: 9 in, 1 out]
      }
      event "Test Slider": Value Change {
        # "When the test mode slider helper is set, update that\ntree row item's value"
        n211 = event-data() -> ("NewVal"=w301:dbl)  [unwired: 1 in]
        n212 = call <vilib>:"NT Write Number.vi"("value"=w301, "name"=w302) -> ()  [unwired: 9 in, 1 out]
      }
      event "On/Off": Value Change {
        # "When the test mode on/off helper value is set, update that\ntree row item's value"
        n213 = event-data() -> ("NewVal"=w305:bool)  [unwired: 1 in]
        n214 = Boolean To (0,1)(Boolean=w305) -> (0, 1=w304:i16)
        n215 = call <vilib>:"NT Write Number.vi"("value"=w304, "name"=w303) -> ()  [unwired: 9 in, 1 out]
      }
      event "Rev/Fwd": Value Change {
        # "When the test mode helper value for relays is set, update that\ntree row item's value"
        n216 = event-data() -> ("NewVal.Forward"=w312:bool, "NewVal.Reverse"=w311:bool)  [unwired: 1 in]
        n217 = Boolean To (0,1)(Boolean=w312) -> (0, 1=w308:i16)
        n218 = Boolean To (0,1)(Boolean=w311) -> (0, 1=w310:i16)
        n219 = Negate(x=w310) -> (-x=w309:i16)
        n220 = Add(x=w308, y=w309) -> (x+y=w307:i16)
        n221 = call <vilib>:"NT Write Number.vi"("value"=w307, "name"=w306) -> ()  [unwired: 9 in, 1 out]
      }
      event "Test Ring": Value Change {
        # "When a test mode helper value is selected from the ring,\nset the tree item's variable to the string value"
        n222 = event-data() -> ("NewVal"=w315:u16)  [unwired: 1 in]
        n223 = property on="Test Ring" class="Ring (strict)"() -> ("Strings []"=w316:string[])  [unwired: 2 in, 2 out]
        n224 = Index Array(array=w316, index=w315) -> (element=w314:string)
        n225 = call <vilib>:"NT Write String.vi"("value"=w314, "name"=w313) -> ()  [unwired: 9 in, 1 out]
      }
      event "Rec Mode": Value Change {
        # "Update globals for recording mode and path to read log from.\nClear when logging and let NetworkTables set path for vision to\nuse."
        n226 = event-data() -> ("NewVal"=w325:enum32{"Stop", "Record", "Playback"})  [unwired: 1 in]
        n227 = global write "WPI_DashboardLogging Global.vi" "Logging Filename"(path "") -> ()
        n228 = global write "WPI_DashboardLogging Global.vi" "Recording"(w325) -> ()
        n229 = case shown="\"Playback\"" w325 {
          tunnel: w324 -> [_ w327 w335]
          tunnel: [_ _ w334] -> w322
          tunnel: [_ _ w333] -> _
          tunnel: w320 -> [_ _ w331]
          tunnel: cluster{i32, i32} {-250, 170} -> [_ _ w330]
          tunnel: [_ _ T19 {"Image Size"=TRUE, "Image Type"=TRUE, "Pixel Value"=TRUE, "ROI Information"=TRUE, "Zoom Factor"=FALSE} ("Image Information Shown:All Elements")] -> w317
          tunnel: [_ _ TRUE ("Zoom Factor")] -> w318
          frame Default {
          }
          frame "Stop", "Record" {
            # "Place Window too"
            n230 = invoke class="VI" method="FP.Close"(reference=w327) -> (reference out=w326:refnum<vi>)  [unwired: 2 in, 2 out]
            n231 = invoke class="VI" method="Abort VI"(reference=w326) -> ()  [unwired: 2 in, 3 out]
          }
          frame "Playback" {
            n232 = call "Open Playback Panel.vi"("Offset"=w330, "DB VI Ref"=w331, "Playback in"=w335) -> ("Playback out"=w332:refnum<vi>)  [unwired: 8 in]
            n233 = register-events(w332) -> (reference out=w334:refnum<event-registration>, error out=w333:errorcluster)  [unwired: 2 in]
          }
        }
        n234 = property on="Camera Image Right" class="ImageControl"("Image Information Shown"=w317, "Image Information Visible"=w318) -> ()  [unwired: 2 in, 2 out]
        n235 = property on="Camera Image" class="ImageControl"("Image Information Shown"=w317, "Image Information Visible"=w318) -> ()  [unwired: 2 in, 2 out]
        n236 = call <vilib>:"WPI_DashboardNT Log FieldName Cache.vi"("Operation"=enum16{"Lookup/Add", "Index", "Clear"}."Clear") -> ()  [unwired: 8 in, 3 out]
      }
      event Panel Close {
        w336 = enum32{"Stop", "Record", "Playback"}."Stop" ("Rec Mode")
        # "Playback window has been closed, abort"
        n237 = event-data() -> ()  [unwired: 1 in, 4 out]
        n238 = local write "Rec Mode"(w336) -> ()
        n239 = global write "WPI_DashboardLogging Global.vi" "Recording"(w336) -> ()
      }
      event Panel Close {
        # "Abort playback window and ourself"
        n240 = event-data() -> ()  [unwired: 1 in, 4 out]
        n241 = invoke class="VI" method="FP.Close"(reference=w339) -> (reference out=w338:refnum<vi>)  [unwired: 2 in, 2 out]
        n242 = invoke class="VI" method="Abort VI"(reference=w338) -> (error out=w337:errorcluster)  [unwired: 2 in, 2 out]
        n243 = invoke class="VI" method="Abort VI"(error in=w337) -> ()  [unwired: 2 in, 3 out]
      }
      event "Tree": Double Click {
        n244 = event-data() -> ("PlatMods"=w345:T21, "Tag"=w342:string)  [unwired: 1 in]
        n245 = Unbundle(w345) -> ("Shift"=w344:bool)  [unwired: 4 out]
        n246 = String Subset(string=w342, length (rest)=1 ("length (rest)")) -> (substring=w341:string)  [unwired: 1 in]
        n247 = Not(x=w344) -> (.not. x?=w343:bool)
        n248 = case shown="\"/\"" w341 {
          tunnel: w342 -> [_ w347]
          tunnel: w343 -> [_ w346]
          frame Default {
          }
          frame "/" {
            n249 = call <vilib>:"NT Update Persistence.vi"("Persistence"=w346, "Name"=w347) -> ()  [unwired: 9 in, 1 out]
          }
        }
      }
    }
  }
  n250 = while {
    tunnel: w61 -> [w349]
    i -> [w352]
    stop <- FALSE stop-if-true
    n251 = Wait (ms)(milliseconds to wait=u32 100) -> ()  [unwired: 1 out]
    n252 = case shown="\"Playback\"" "Rec Mode" {
      tunnel: w352 -> [_ _ w367]
      tunnel: [u32 2829099 ("Base Color") u32 11141120 ("Target Color") w356] -> w348
      frame "Stop", Default {
        # "Reset the color, extra updates don't cost much"
      }
      frame "Record" {
      }
      frame "Playback" {
        # "Playback"
        n253 = Quotient & Remainder(x=w367, y=u32 50 ("milliseconds to wait")) -> (x-y*floor(x/y)=w363:u32)  [unwired: 1 out]
        n254 = Divide(x=w363, y=u32 50 ("milliseconds to wait")) -> (x/y=w360:dbl)
        n255 = Multiply(x=6.283185307179586, y=w360) -> (x*y=w365:dbl)
        n256 = Sine(x=w365) -> (sin(x)=w364:dbl)
        n257 = Absolute Value(x=w364) -> (abs(x)=w357:dbl)
        n258 = call "Interpolate RGB Color.vi"("Proportion"=w357, "Target Color"=u32 30976, "Base Color"=u32 2829099) -> ("Result Color"=w356:u32)  [unwired: 8 in]
      }
    }
    n259 = property class="Pane"(reference=w349, "PaneColor"=w348) -> ()  [unwired: 1 in, 2 out]
  }
  n260 = local write "Dashboard Tab"(T3."Drive" ("Dashboard Tab")) -> ()
  n261 = control-ref of="Field Picture"() -> (w4:refnum<vi>)
  n262 = control-ref of="ROBOT"() -> (w5:refnum<vi>)
  n263 = property on="On/Off" class="Bool (strict)"("Visible"=w34) -> ()  [unwired: 2 in, 2 out]
  n264 = property on="Motor" class="Clust (strict)"("Visible"=w34) -> ()  [unwired: 2 in, 2 out]
  n265 = property on="Progress" class="Clust (strict)"("Visible"=w34) -> ()  [unwired: 2 in, 2 out]
  n266 = property on="Test Ring" class="Ring (strict)"("Visible"=w34) -> ()  [unwired: 2 in, 2 out]
  n267 = property on="Rev/Fwd" class="Clust (strict)"("Visible"=w34) -> ()  [unwired: 2 in, 2 out]
  n268 = while {
    tunnel: u16 1741 ("timeout ms (25000)") -> [w369]
    stop <- FALSE stop-if-true
    n269 = TCP Create Listener(10:w369) -> (0:w368:errorcluster, 3:w370:refnum<k5>)  [unwired: 4 in, 1 out]
    n270 = case shown="No Error" w368 {
      selector: w368 -> [w372 _]
      tunnel: w370 -> [w373 _]
      frame No Error {
        n271 = while {
          tunnel: w373 -> [w376]
          tunnel: w372 -> [w375]
          stop <- FALSE stop-if-true
          n272 = TCP Wait On Listener(8:w375, 11:w376) -> (0:w377:errorcluster, 4:w378:refnum<k5>)  [unwired: 2 in, 3 out]
          n273 = local write "TCP"(w378) -> ()
          n274 = case shown="Error" w377 {
            frame No Error {
            }
            frame Error {
              n275 = Wait (ms)(milliseconds to wait=u32 1000) -> ()  [unwired: 1 out]
            }
          }
        }
      }
      frame Error {
        n276 = Wait (ms)(milliseconds to wait=u32 1000) -> ()  [unwired: 1 out]
      }
    }
  }
  n277 = call <vilib>:"FieldDisp_Field_Disp.vi"("Field Selector"="2024 Crescendo Miklast", "Picture in"=w4) -> ("error out"=w7:errorcluster)  [unwired: 9 in]
  n278 = call <vilib>:"FieldDisp_Element_Prepare.vi"("Element File Name"="Robot_kitbot_5.png" ("Picture FIle Name"), "Element Picture Ref"=w5, "Field Picture Ref"=w4) -> ("error out"=w2:errorcluster, "Field Element Info"=w3:T22)  [unwired: 7 in]
  n279 = while {
    tunnel: [w391] -> _
    tunnel: w33 -> [w383]
    tunnel: w7 -> [w382]
    tunnel: w3 -> [w381]
    i -> [w391]
    stop <- FALSE stop-if-true
    n280 = call <vilib>:"WPI_DashboardRetrieveStatusInfo.vi"("Window Mode Notifier"=w383, "TCP Cnx"="TCP") -> ("Power and Errors"=w386:T24, "Robot Metrics"=w389:T25, "Status Info"=w390:T26, "Control Info"=w387:T27, "Robot Mode"=w385:T5, "Process?"=w388:bool)  [unwired: 4 in]
    "Mode" <- w385
    n281 = case shown="True" w388 {
      tunnel: w390 -> [_ w533]
      tunnel: w389 -> [_ w532]
      tunnel: w387 -> [_ w531]
      tunnel: w386 -> [_ w530]
      tunnel: w385 -> [_ _]
      tunnel: w382 -> [_ _]
      tunnel: w381 -> [_ w440]
      frame False {
        n282 = Wait (ms)(milliseconds to wait=u32 20) -> ()  [unwired: 1 out]
      }
      frame True {
        w405 = T23."Drive" ("x")
        # "tab changed."
        # "y"
        # "x"
        # "Auto"
        # "Climb"
        # "Arm"
        # "Box"
        # "Arm"
        n283 = Unbundle By Name(w531) -> ("Joystick Values"=w529:T28)  [unwired: 1 out]
        n284 = Unbundle By Name(w532) -> ()  [unwired: 1 out]
        n285 = Unbundle By Name(w530) -> ("Robot IP"=→"Robot IP":string)
        n286 = Unbundle By Name(w533) -> ()  [unwired: 2 out]
        n287 = call-poly <vilib>:"NT Read Value.vi"("name"="Vision/Xcurrent in feet") -> ("value"=w421:dbl)  [unwired: 8 in, 2 out]
        "Robot X" <- w421
        n288 = call-poly <vilib>:"NT Read Value.vi"("name"="Vision/Y current in feet") -> ("value"=w420:dbl)  [unwired: 8 in, 2 out]
        "Robot Y" <- w420
        n289 = call-poly <vilib>:"NT Read Value.vi"("name"="Vision/angle current") -> ("value"=w422:dbl)  [unwired: 8 in, 2 out]
        "Robot Angle" <- w422
        n290 = call-poly <vilib>:"NT Read Value.vi"("name"="Arm/LiftForwardLimit") -> ("value"=→"Lower Limit Switch":bool)  [unwired: 8 in, 2 out]
        n291 = call-poly <vilib>:"NT Read Value.vi"("name"="Arm/LiftDemand") -> ("value"=w511:dbl)  [unwired: 8 in, 2 out]
        "SP Deg" <- w511
        n292 = call-poly <vilib>:"NT Read Value.vi"("name"="Arm/LiftSensorPosition") -> ("value"=w510:dbl)  [unwired: 8 in, 2 out]
        "PV Deg" <- w510
        n293 = call-poly <vilib>:"NT Read Value.vi"("name"="Arm/LiftSensorVelocity") -> ("value"=w508:dbl)  [unwired: 8 in, 2 out]
        "Velocity Deg/Sec" <- w508
        n294 = call-poly <vilib>:"NT Read Value.vi"("name"="Arm/MotorOutput") -> ("value"=w509:dbl)  [unwired: 8 in, 2 out]
        "CO" <- w509
        n295 = call-poly <vilib>:"NT Read Value.vi"("name"="Arm/OnTarget") -> ("value"=→"Arm on Target":bool)  [unwired: 8 in, 2 out]
        n296 = call <vilib>:"Conv_Feet_Meters.vi"("Feet"=w421) -> ("Meters"=w443:dbl)  [unwired: 10 in]
        n297 = call <vilib>:"Conv_Feet_Meters.vi"("Feet"=w420) -> ("Meters"=w442:dbl)  [unwired: 10 in]
        n298 = call <vilib>:"Conv_Deg_Radians.vi"("Degress"=w422) -> ("Radians"=w441:dbl)  [unwired: 10 in]
        n299 = Bundle("value"=w511, "value"=w510, "value"=w509, "value"=w508) -> (→"Arm Chart":T7)  [unwired: 1 in]
        n300 = Index Array(array=w529) -> (element #1=w528:T29, element #2=w524:T29)  [unwired: 2 in]
        n301 = call "Prepare Joystick Data for Displays.vi"("Joystick Values"=w524) -> ("Buttons"=→"JS2 Buttons":T30, "Z Axis"=→"JS2 Z":dbl, "Cartesian Data"=→"JS2 Graph":cluster{"X axis":dbl, "X axis":dbl}[])  [unwired: 8 in]
        n302 = call "Prepare Joystick Data for Displays.vi"("Joystick Values"=w528) -> ("Buttons"=→"JS1 Buttons":T30, "Z Axis"=→"JS1 Z":dbl, "Cartesian Data"=→"JS1 Graph":cluster{"X axis":dbl, "X axis":dbl}[])  [unwired: 8 in]
        n303 = Equal?(x=w405, y=T23."Field") -> (x = y?=w438:bool)
        n304 = feedback #1(T23."Drive" ("Dashboard Tab")) -> (w437:T23)
        n305 = feedback-in #1(w405) -> ()
        n306 = Not Equal?(x=w405, y=w437) -> (x != y?=w436:bool)
        n307 = case shown="True" w438 {
          tunnel: w440 -> [w557 w562]
          tunnel: w441 -> [_ w565]
          tunnel: w443 -> [_ w564]
          tunnel: w442 -> [_ w563]
          tunnel: w436 -> [w556 w561]
          frame False {
            n308 = case shown="True" w556 {
              tunnel: w557 -> [_ w558]
              frame False {
              }
              frame True {
                n309 = Unbundle By Name(w558) -> ("Element Picture Ref"=w559:refnum<vi>)
                n310 = property class="Pict"(reference=w559, "Visible"=FALSE) -> ()  [unwired: 1 in, 2 out]
              }
            }
          }
          frame True {
            # "Update display\nof field element\n(robot)"
            n311 = call <vilib>:"Pose2d_New.vi"("Heading"=w565, "Y"=w563, "X"=w564) -> ("out POSe"=w566:T31)  [unwired: 8 in]
            n312 = call <vilib>:"FieldDisp_Element_Disp.vi"("Element Pose"=w566, "Element Info"=w562) -> ()  [unwired: 10 in]
            n313 = case shown="True" w561 {
              tunnel: w562 -> [_ w567]
              frame False {
              }
              frame True {
                n314 = Unbundle By Name(w567) -> ("Element Picture Ref"=w568:refnum<vi>)
                n315 = property class="Pict"(reference=w568, "Visible"=TRUE) -> ()  [unwired: 1 in, 2 out]
              }
            }
          }
        }
        n316 = call-poly <vilib>:"NT Read Value.vi"("name"="Vision/Left vision found count") -> ("value"=w431:dbl)  [unwired: 8 in, 2 out]
        n317 = call-poly <vilib>:"NT Read Value.vi"("name"="Vision/Right vision found count") -> ("value"=w428:dbl)  [unwired: 8 in, 2 out]
        n318 = call-poly <vilib>:"NT Read Value.vi"("name"="Climb/FowardLimitSwitchLeft") -> ("value"=→"Left Upper (Virtual) Limit":bool)  [unwired: 8 in, 2 out]
        n319 = call-poly <vilib>:"NT Read Value.vi"("name"="Climb/Demand") -> ("value"=w486:dbl)  [unwired: 8 in, 2 out]
        "SP Inches" <- w486
        n320 = call-poly <vilib>:"NT Read Value.vi"("name"="Climb/RevLimLeft") -> ("value"=→"Left Low Limit" →"Left Limit":bool)  [unwired: 8 in, 2 out]
        n321 = call-poly <vilib>:"NT Read Value.vi"("name"="Climb/SensorPosLeft") -> ("value"=w485:dbl)  [unwired: 8 in, 2 out]
        "Left PV" <- w485
        n322 = call-poly <vilib>:"NT Read Value.vi"("name"="Climb/SensorVelocityLeft") -> ("value"=→"Left Vel":dbl)  [unwired: 8 in, 2 out]
        n323 = feedback #2() -> (w430:dbl)  [unwired: 1 in]
        n324 = feedback-in #2(w431) -> ()
        n325 = call-poly <vilib>:"NT Read Value.vi"("name"="Climb/MotorOutLeft") -> ("value"=w483:dbl)  [unwired: 8 in, 2 out]
        "Left Co" <- w483
        n326 = feedback #3() -> (w427:dbl)  [unwired: 1 in]
        n327 = feedback-in #3(w428) -> ()
        n328 = call-poly <vilib>:"NT Read Value.vi"("name"="Climb/OnTargetLeft") -> ("value"=→"Left On Targ":bool)  [unwired: 8 in, 2 out]
        n329 = call-poly <vilib>:"NT Read Value.vi"("name"="Vision/Left vision connect") -> ("value"=→"Left Cam Connected":bool)  [unwired: 8 in, 2 out]
        n330 = call-poly <vilib>:"NT Read Value.vi"("name"="Vision/Right vision connect") -> ("value"=→"Right Cam Connected":bool)  [unwired: 8 in, 2 out]
        n331 = Not Equal?(x=w431, y=w430) -> (x != y?=→"Left April Tag Updated":bool)
        n332 = Not Equal?(x=w428, y=w427) -> (x != y?=→"Right April Tag Updated":bool)
        n333 = call-poly <vilib>:"NT Read Value.vi"("name"="Shooter/RshooterSpeed") -> ("value"=w448:dbl)  [unwired: 8 in, 2 out]
        "R Speed" <- w448
        n334 = call-poly <vilib>:"NT Read Value.vi"("name"="Shooter/Future") -> ("value"=w447:dbl)  [unwired: 8 in, 2 out]
        "R Mot" <- w447
        n335 = call-poly <vilib>:"NT Read Value.vi"("name"="Shooter/Future") -> ("value"=w449:dbl)  [unwired: 8 in, 2 out]
        "L Mot" <- w449
        n336 = call-poly <vilib>:"NT Read Value.vi"("name"="Climb/FowardLimitSwitchRight") -> ("value"=→"Right Upper (Virtual) Limit":bool)  [unwired: 8 in, 2 out]
        n337 = call-poly <vilib>:"NT Read Value.vi"("name"="Climb/RevLimRight") -> ("value"=→"Right Low Limit" →"Right Limit":bool)  [unwired: 8 in, 2 out]
        n338 = call-poly <vilib>:"NT Read Value.vi"("name"="Climb/SensorPosRight") -> ("value"=w484:dbl)  [unwired: 8 in, 2 out]
        "Right PV" <- w484
        n339 = call-poly <vilib>:"NT Read Value.vi"("name"="Climb/SensorVelocityRight") -> ("value"=→"Right Vel":dbl)  [unwired: 8 in, 2 out]
        n340 = call-poly <vilib>:"NT Read Value.vi"("name"="Climb/MotorOutRight") -> ("value"=w482:dbl)  [unwired: 8 in, 2 out]
        "Right Co" <- w482
        n341 = call-poly <vilib>:"NT Read Value.vi"("name"="Climb/OnTargetRight") -> ("value"=→"Right On Targ":bool)  [unwired: 8 in, 2 out]
        n342 = call-poly <vilib>:"NT Read Value.vi"("name"="Shooter/LshooterSpeed") -> ("value"=w450:dbl)  [unwired: 8 in, 2 out]
        "L Speed" <- w450
        n343 = call-poly <vilib>:"NT Read Value.vi"("name"="Shooter/Future") -> ("value"=w451:dbl)  [unwired: 8 in, 2 out]
        "Shoot SP\nRPM" <- w451
        n344 = Bundle("value"=w451, "value"=w450, "value"=w449, "value"=w448, "value"=w447) -> (→"Shoot Chart":T8)  [unwired: 1 in]
        n345 = Bundle("value"=w486, "value"=w485, "value"=w484, "value"=w483, "value"=w482) -> (→"Climb Chart":T8)  [unwired: 1 in]
        n346 = disable-structure shown="Disabled" {
          frame Disabled {
            n347 = call-poly <vilib>:"NT Read Value.vi"("name"="Boolean") -> ("value"=w534:dbl)  [unwired: 8 in, 2 out]
            n348 = call-poly <vilib>:"NT Read Value.vi"("name"="Boolean") -> ("value"=w546:bool)  [unwired: 8 in, 2 out]
            n349 = call-poly <vilib>:"NT Read Value.vi"("name"="Boolean") -> ("value"=w539:bool)  [unwired: 8 in, 2 out]
            n350 = call-poly <vilib>:"NT Read Value.vi"("name"="Boolean") -> ("value"=w538:bool)  [unwired: 8 in, 2 out]
            n351 = call-poly <vilib>:"NT Read Value.vi"("name"="Boolean") -> ("value"=w537:bool)  [unwired: 8 in, 2 out]
            n352 = call-poly <vilib>:"NT Read Value.vi"("name"="Boolean") -> ("value"=w536:bool)  [unwired: 8 in, 2 out]
            n353 = call-poly <vilib>:"NT Read Value.vi"("name"="Boolean") -> ("value"=w540:bool)  [unwired: 8 in, 2 out]
          }
          frame Enabled {
          }
        }
        n354 = call-poly <vilib>:"NT Read Value.vi"("name"="Arm/CalcSpeaker_Enabled") -> ("value"=→"Auto Arm":bool)  [unwired: 8 in, 2 out]
        n355 = call-poly <vilib>:"NT Read Value.vi"("name"="Arm/LiftDemand") -> ("value"=→"Demand":dbl)  [unwired: 8 in, 2 out]
        n356 = call-poly <vilib>:"NT Read Value.vi"("name"="Arm/LiftSensorPosition") -> ("value"=→"Position":dbl)  [unwired: 8 in, 2 out]
        n357 = call-poly <vilib>:"NT Read Value.vi"("name"="Arm/OnTarget") -> ("value"=→"On Target":bool)  [unwired: 8 in, 2 out]
        n358 = call-poly <vilib>:"NT Read Value.vi"("name"="Auto/Selected") -> ("value"=→"Selected Auto":string)  [unwired: 8 in, 2 out]
        n359 = call-poly <vilib>:"NT Read Value.vi"("name"="Climb/Demand") -> ("value"=→"Dmd":dbl)  [unwired: 8 in, 2 out]
        n360 = call-poly <vilib>:"NT Read Value.vi"("name"="Climb/SensorPosLeft") -> ("value"=→"Left\nPosition":dbl)  [unwired: 8 in, 2 out]
        n361 = call-poly <vilib>:"NT Read Value.vi"("name"="Climb/SensorPosRight") -> ("value"=→"Right\nPosition":dbl)  [unwired: 8 in, 2 out]
        n362 = call-poly <vilib>:"NT Read Value.vi"("name"="Boolean") -> ("value"=→"Climb Blocked":bool)  [unwired: 8 in, 2 out]
        n363 = call-poly <vilib>:"NT Read Value.vi"("name"="Climb/Demand") -> ("value"=→"Dmd 2":dbl)  [unwired: 8 in, 2 out]
        n364 = call-poly <vilib>:"NT Read Value.vi"("name"="Climb/SensorPosLeft") -> ("value"=→"Left Pos":dbl)  [unwired: 8 in, 2 out]
        n365 = call-poly <vilib>:"NT Read Value.vi"("name"="Climb/SensorPosRight") -> ("value"=→"Right Pos":dbl)  [unwired: 8 in, 2 out]
        n366 = call-poly <vilib>:"NT Read Value.vi"("name"="Shooter/Box sensor state") -> ("value"=w459:string)  [unwired: 8 in, 2 out]
        n367 = call-poly <vilib>:"NT Read Value.vi"("name"="drive/GryoZ") -> ("value"=w417:dbl)  [unwired: 8 in, 2 out]
        n368 = call-poly <vilib>:"NT Read Value.vi"("name"="Shooter/Box_Ready") -> ("value"=→"Box Ready":bool)  [unwired: 8 in, 2 out]
        n369 = Equal?(x=w459, y="note misaligened") -> (x = y?=→"Misaligned":bool)
        n370 = Equal?(x=w459, y="Has a note") -> (x = y?=→"Have Note":bool)
        n371 = call-poly <vilib>:"NT Read Value.vi"("name"="Shooter/Box sensor state") -> ("value"=→"State":string)  [unwired: 8 in, 2 out]
        n372 = case shown="True" "Update" {
          tunnel: w417 -> [_ w555]
          frame False {
          }
          frame True {
            n373 = Add(x="Rotation", y=w555) -> (x+y=w553:dbl)
            "Int Gyro" <- w553
            n374 = call-poly <vilib>:"NT Write Value.vi"("value"=w553, "name"="drive/IntRobotOrientation") -> ()  [unwired: 9 in, 1 out]
          }
        }
        n375 = call-poly <vilib>:"NT Read Value.vi"("name"="drive/GyroCalibrated") -> ("value"=→"Calibrated":bool)  [unwired: 8 in, 2 out]
        n376 = call-poly <vilib>:"NT Read Value.vi"("name"="drive/IntRobotOrientation_feedback") -> ("value"=→"Int Gyro Feedback":dbl)  [unwired: 8 in, 2 out]
        n377 = call-poly <vilib>:"NT Write Value.vi"("value"="Calibrate", "name"="drive/CalGyro") -> ()  [unwired: 9 in, 1 out]
        n378 = case shown="True" "Intake Update" {
          tunnel: "Intake" -> [_ w548]
          frame False {
          }
          frame True {
            n379 = call-poly <vilib>:"NT Write Value.vi"("value"=w548, "name"="Box/IntakeGetMotorDMD") -> ()  [unwired: 9 in, 1 out]
          }
        }
        n380 = case shown="True" "Shoot Update" {
          tunnel: "Shoot Speed" -> [_ w550]
          frame False {
          }
          frame True {
            n381 = call-poly <vilib>:"NT Write Value.vi"("value"=w550, "name"="Box/ShooterSpeedRPM") -> ()  [unwired: 9 in, 1 out]
          }
        }
      }
    }
  }
  n382 = global write "WPI_DashboardLogging Global.vi" "Recording"(w56) -> ()
  n383 = local write "Rec Mode"(w56) -> ()
  n384 = call <vilib>:"NT Write String.vi"("value"="Select Auto", "name"="Auto Selector" ("Name")) -> ()  [unwired: 9 in, 1 out]
  n385 = case shown="Error .." w2 {
    frame No Error {
    }
    frame Error {
      n386 = One Button Dialog(message="Could not read robot image.") -> ()  [unwired: 1 in, 1 out]
    }
  }
